vi "Low Limit is null.vi"(8 "error in":errorcluster, 11 "Sub Object in":refnum<class "Sub Object.lvclass">) -> (0 "error out":errorcluster, 2 "Null":bool=TRUE, 3 "Sub Object out":refnum<class "Sub Object.lvclass">)   [LabVIEW 2020, in "CANopen.lvlib" / "Sub Object.lvclass"]
uses:
  Sub Object.lvclass
  Sub Object.lvclass/Sub Object.ctl
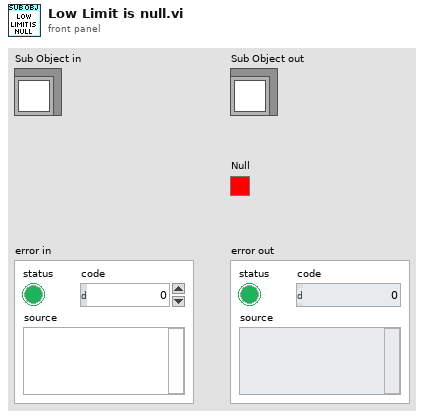
[diagram p1: front panel]
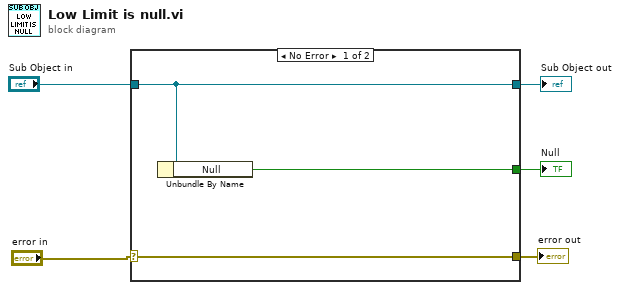
[diagram p0: block diagram]
diagram:
  n1 = case shown="No Error" "error in" {
    selector: "error in" -> [w8 w9]
    tunnel: [w8 w9] -> w2
    tunnel: [w7 w10] -> w4
    tunnel: "Sub Object in" -> [w7 w10]
    tunnel: [w6 _] -> w1
    frame No Error {
      n2 = Unbundle By Name(w7) -> ("Null"=w6:bool)
    }
    frame Error {
    }
  }
  "error out" <- w2
  "Sub Object out" <- w4
  "Null" <- w1
